vi "Dresser DXD Delay n mSec.vi"(0 "VISA session":refnum<visa-resource-name>, 1 "Milliseconds to Wait (0)":u32, 11 "Error In (no error)":errorcluster) -> (4 "dup VISA session":refnum<visa-resource-name>, 15 "Error Out":errorcluster)   [LabVIEW 2015]
doc: "This VI will read the first 160 bytes of EEPROM memory of the Dresser DXD Series pressure transducer, as a string of decimal values. The raw string returned is formatted with 16 bytes per line with carriage return/line feeds appended at ends. The raw string is converted to an array of digital numbers for ease of indexing to a location. Index 0 corresponds to byte 0, index 1 corresponds to byte 1, etc.\n\nWritten by:\nBLOOMY CONTROLS, INC\nWINDSOR, CT 06095, USA\n860-298-9925\nwww.bloomy.com\nV2.0.0\nMay, 2002"
panel:
  # "For instructions on the use of this VI, press Ctrl+H to display the help window and move the mouse over the icon, controls, and indicators"
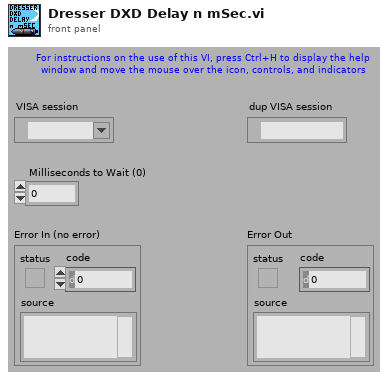
[diagram p1: front panel]
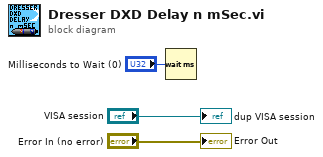
[diagram p0: block diagram]
diagram:
  n1 = Wait (ms)(milliseconds to wait="Milliseconds to Wait (0)") -> ()  [unwired: 1 out]
  "Error Out" <- "Error In (no error)"
  "dup VISA session" <- "VISA session"
